vi "Initialize Tag Tree.vi"(8 "error in (no error)":errorcluster, 10 "Tag Tree Helper":refnum<class "Tag Tree Helper.lvclass">, 11 "New Class Dialog In":refnum<class "New Class Dialog.lvclass">) -> (0 "error out":errorcluster, 3 "New Class Dialog Out":refnum<class "New Class Dialog.lvclass">)   [LabVIEW 2020, in "New Class Dialog.lvclass"]
uses:
  New Class Dialog.lvclass
  Helpers/Tag Tree Helper/Tag Tree Helper.lvclass
  New Class Dialog.lvclass/New Class Dialog.ctl
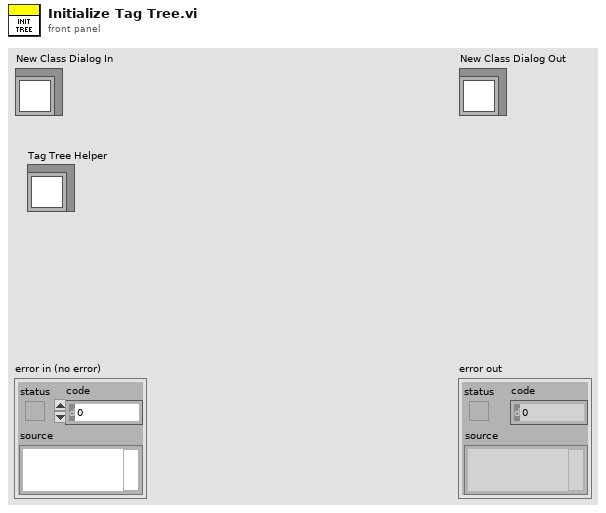
[diagram p1: front panel]
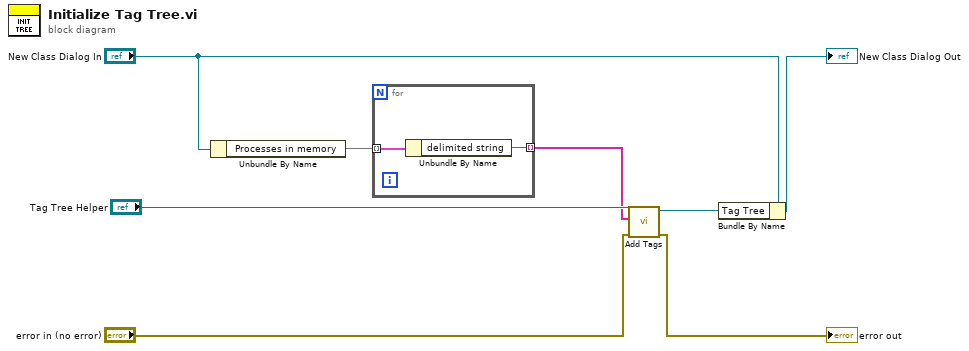
[diagram p0: block diagram]
diagram:
  n1 = Unbundle By Name("New Class Dialog In") -> ("Processes in memory"=w7:map{string, path})
  n2 = for {
    tunnel: w7 -> [w10] mode=indexing
    tunnel: [w9] -> w5 mode=indexing
    n3 = Unbundle By Name(w10) -> ("delimited string"=w9:string)
  }
  n4 = call "Add Tags.vi"("error in (no error)"="error in (no error)", "Tag"=w5, "Tag Tree Helper In"="Tag Tree Helper") -> ("error out"=→"error out":errorcluster, "Tag Tree Helper Out"=w3:refnum<class "Tag Tree Helper.lvclass">)  [unwired: 7 in]
  n5 = Bundle By Name(cluster="New Class Dialog In", "Tag Tree"=w3) -> (→"New Class Dialog Out":refnum<class "New Class Dialog.lvclass">)
